vi "HTTP_GET_Test_Arduino_AddData.vi"(8 "error in (no error)":errorcluster, 9 "userdata=":string, 11 "reqnum":string) -> (0 "error out":errorcluster, 3 "body":string)   [LabVIEW 2017]
panel:
  out "concatenated string":string
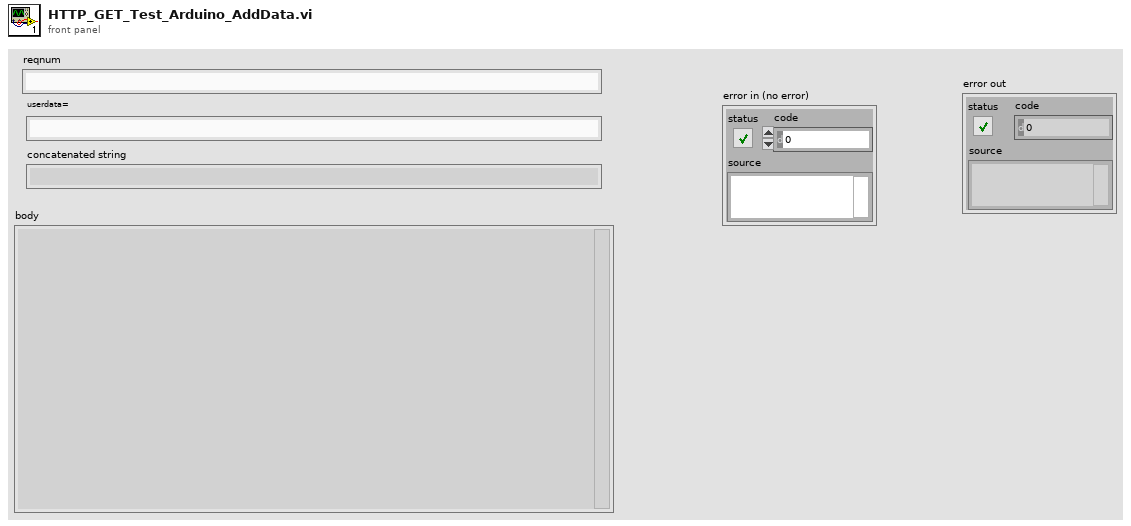
[diagram p1: front panel]
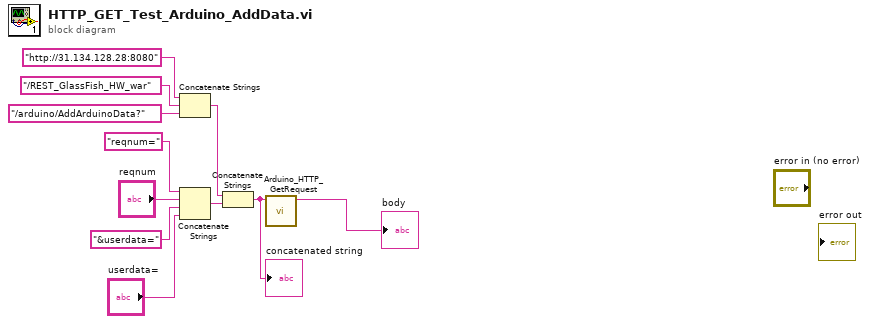
[diagram p0: block diagram]
diagram:
  n1 = Concatenate Strings("http://31.134.128.28:8080" ("url"), "/REST_GlassFish_HW_war" ("url"), "/arduino/AddArduinoData?" ("url")) -> (w8:string)
  n2 = Concatenate Strings("reqnum=" ("url"), "reqnum", "&userdata=" ("url"), "userdata=") -> (w7:string)
  n3 = Concatenate Strings(w8, w7) -> (w2:string)
  "concatenated string" <- w2
  n4 = call <vilib>:"Arduino_HTTP_GetRequest.vi"("Request string"=w2) -> ("body"=→"body":string)  [unwired: 9 in, 1 out]
